vi "ConfigRefClkSource.vi"(8 "error in (no error)":errorcluster, 11 "ClassIn":refnum<class "NiPxi6733.lvclass">) -> (0 "error out":errorcluster, 3 "ClassOut":refnum<class "NiPxi6733.lvclass">)   [LabVIEW 2014, in "FGenPlugins.lvlib" / "NiPxi6733.lvclass"]
uses:
  NiPxi6733.lvclass
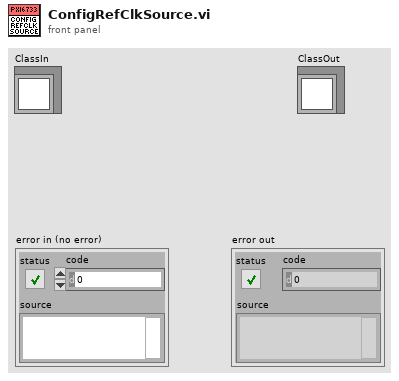
[diagram p1: front panel]
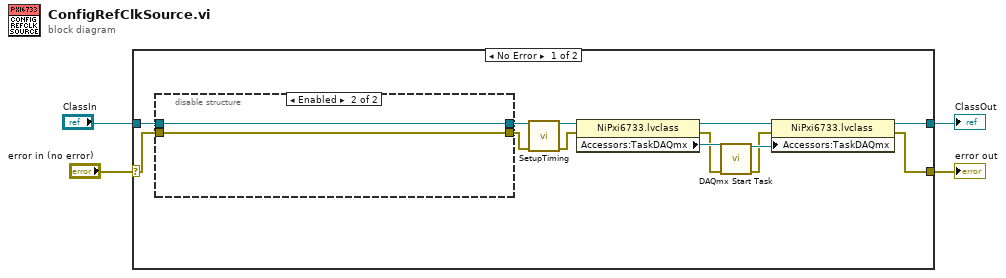
[diagram p0: block diagram]
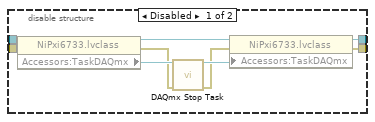
[diagram p2: hidden frame]
diagram:
  n1 = case shown="No Error" "error in (no error)" {
    selector: "error in (no error)" -> [w16 w29]
    tunnel: "ClassIn" -> [w17 w30]
    tunnel: [w8 w30] -> w1
    tunnel: [w5 w29] -> w2
    frame No Error {
      n2 = disable-structure shown="Enabled" {
        disable-tunnel: w17 -> [w26 w28]
        disable-tunnel: w16 -> [w24 w27]
        disable-tunnel: [w21 w28] -> w14
        disable-tunnel: [w18 w27] -> w13
        frame Disabled {
          n3 = property class="NiPxi6733.lvclass"(reference=w26, error in=w24) -> (reference out=w22:refnum<class "NiPxi6733.lvclass">, error out=w23:errorcluster, "Accessors:TaskDAQmx"=w25:refnum<k21>)
          n4 = call <vilib>:"DAQmx Stop Task.vi"("task/channels in"=w25, "error in"=w23) -> ("task out"=w20:refnum<k21>, "error out"=w19:errorcluster)  [unwired: 12 in]
          n5 = property class="NiPxi6733.lvclass"(reference=w22, error in=w19, "Accessors:TaskDAQmx"=w20) -> (reference out=w21:refnum<class "NiPxi6733.lvclass">, error out=w18:errorcluster)
        }
        frame Enabled {
        }
      }
      n6 = call "SetupTiming.vi"("error in (no error)"=w13, "ClassIn"=w14) -> ("error out"=w11:errorcluster, "ClassOut"=w15:refnum<class "NiPxi6733.lvclass">)  [unwired: 8 in]
      n7 = property class="NiPxi6733.lvclass"(reference=w15, error in=w11) -> (reference out=w12:refnum<class "NiPxi6733.lvclass">, error out=w9:errorcluster, "Accessors:TaskDAQmx"=w10:refnum<k21>)
      n8 = call <vilib>:"DAQmx Start Task.vi"("task/channels in"=w10, "error in"=w9) -> ("task out"=w7:refnum<k21>, "error out"=w6:errorcluster)  [unwired: 12 in]
      n9 = property class="NiPxi6733.lvclass"(reference=w12, error in=w6, "Accessors:TaskDAQmx"=w7) -> (reference out=w8:refnum<class "NiPxi6733.lvclass">, error out=w5:errorcluster)
    }
    frame Error {
    }
  }
  "error out" <- w2
  "ClassOut" <- w1
